vi "Get Channel Wise Calibration parameters.vi"(8 "error in (no error)":errorcluster, 10 "Physical Cgannel":string[](array[string]), 11 "Calibration Table":string[][](array[string])) -> (0 "error out":errorcluster, 2 "Array 2":sgl[][](array[numeric]), 3 "Slop & Offset":sgl[][](array[numeric]))   [LabVIEW 2018]
panel:
  out "subarray 2":string[](array[string])
  out "subarray":string[](array[string])
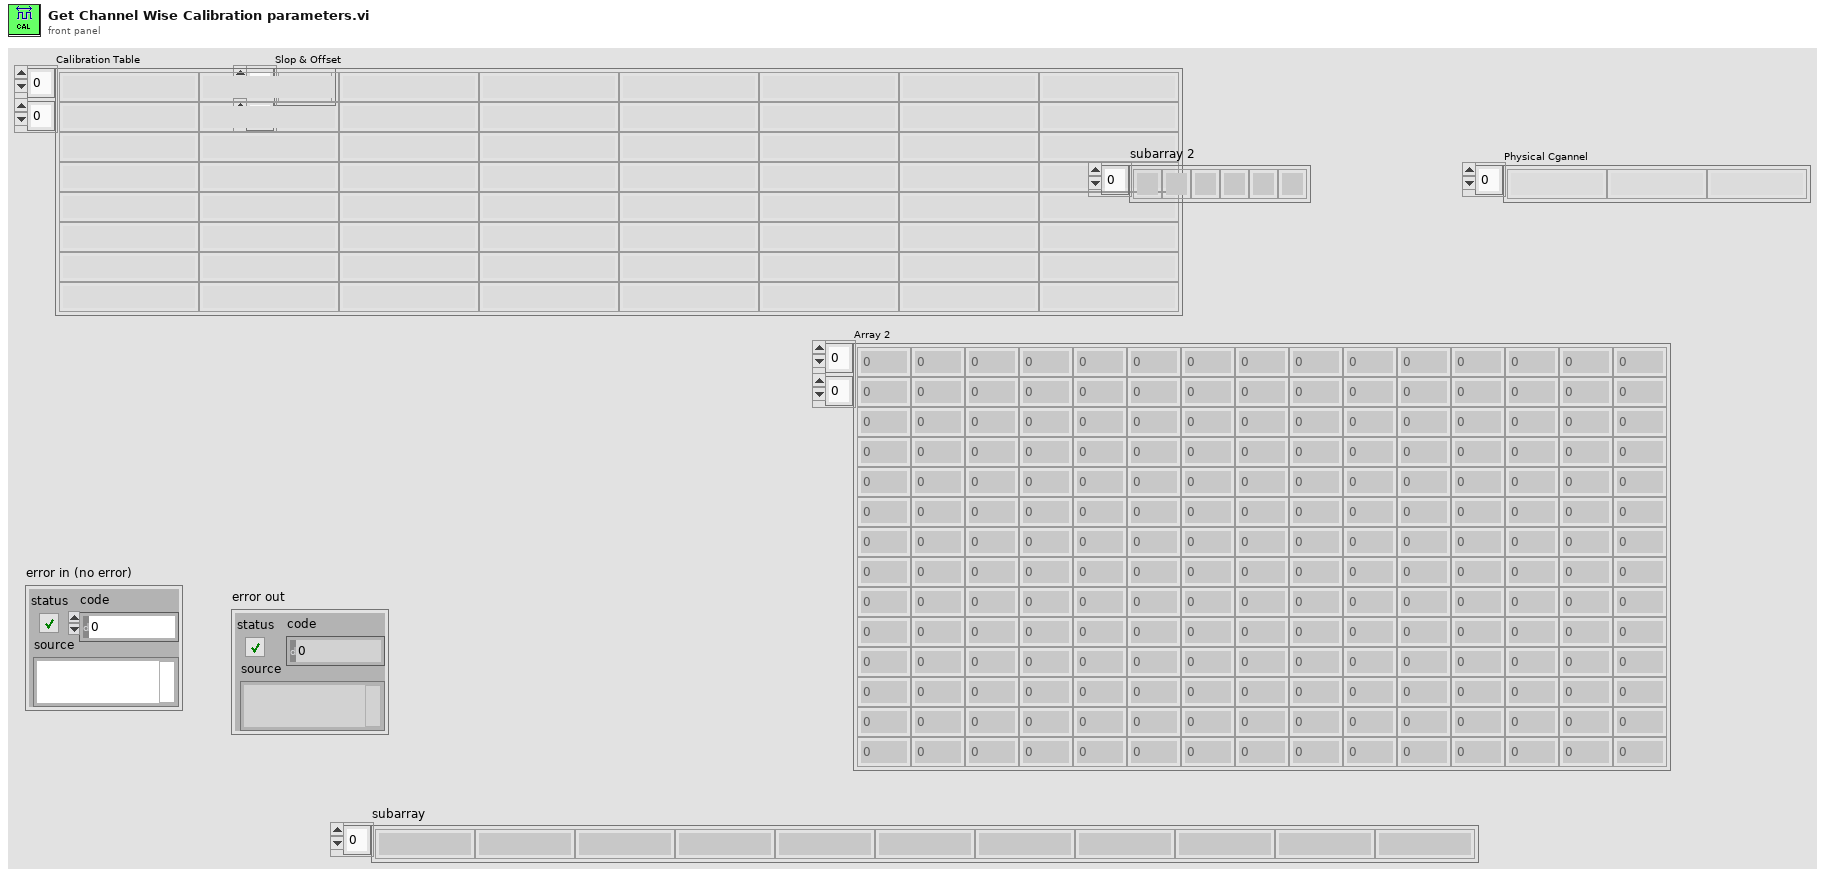
[diagram p1: front panel]
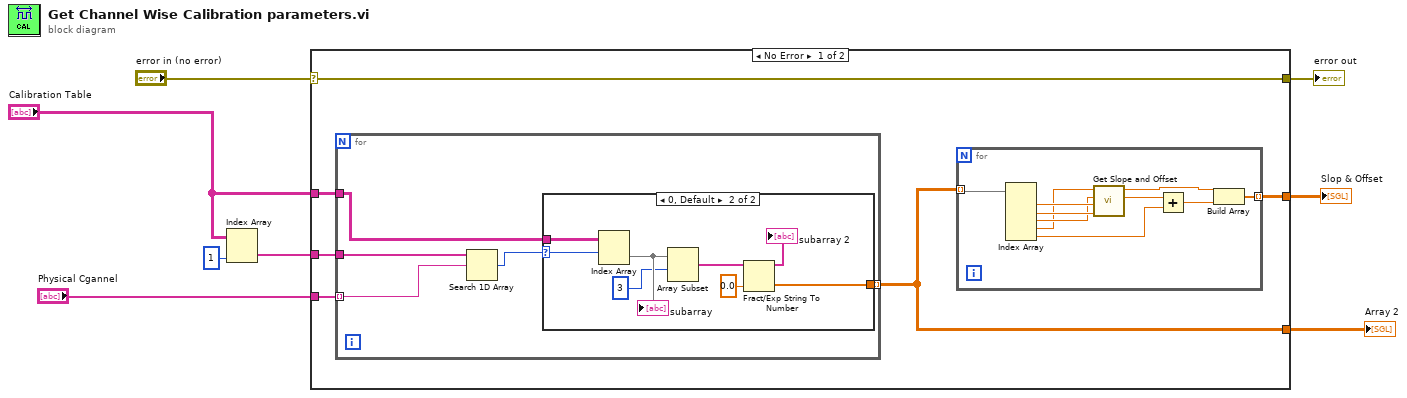
[diagram p0: block diagram]
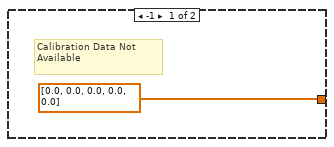
[diagram p2: hidden frame]
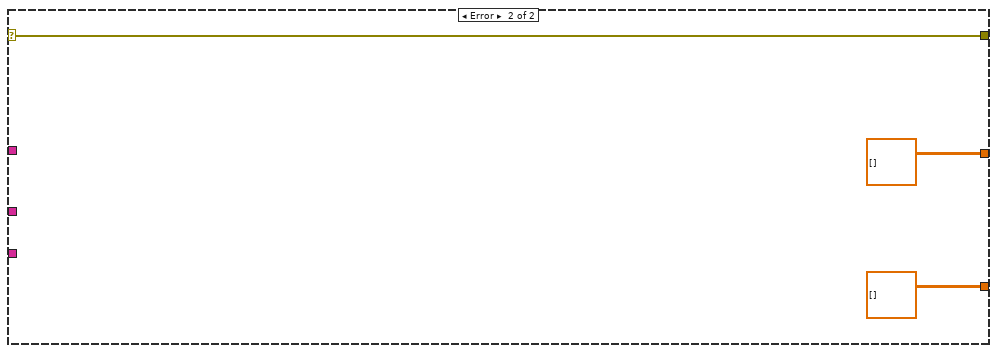
[diagram p3: hidden frame]
diagram:
  n1 = Index Array(array="Calibration Table", index (col)=1 ("disabled index (col)")) -> (element=w4:string[])  [unwired: 1 in]
  n2 = case shown="No Error" "error in (no error)" {
    selector: "error in (no error)" -> [w9 w38]
    tunnel: [w14 sgl[][] []] -> w8
    tunnel: [w13 sgl[][] [] ("Array")] -> w7
    tunnel: "Calibration Table" -> [w12 _]
    tunnel: "Physical Cgannel" -> [w11 _]
    tunnel: w4 -> [w10 _]
    tunnel: [w9 w38] -> w1
    frame No Error {
      n3 = for {
        tunnel: w10 -> [w29]
        tunnel: w11 -> [w28] mode=indexing
        tunnel: w12 -> [w27]
        tunnel: [w26] -> w13 mode=indexing
        n4 = Search 1D Array(1D array=w29, element=w28) -> (index of element=w25:i32)  [unwired: 1 in]
        n5 = case shown="0, Default" w25 {
          selector: w25 -> [_ w31]
          tunnel: w27 -> [_ w37]
          tunnel: [sgl[] [0.0, 0.0, 0.0, 0.0, 0.0] ("Array") w32] -> w26
          frame -1 {
            # "Calibration Data Not \nAvailable"
          }
          frame 0, Default {
            n6 = Index Array "Index Array"(array=w37, index (row)=w31) -> (element=w36:string[])  [unwired: 1 in]
            "subarray" <- w36
            n7 = Array Subset "Array Subset"(array=w36, index=3) -> (w34:string[])  [unwired: 1 in]
            "subarray 2" <- w34
            n8 = Fract/Exp String To Number(string=w34, default (0 dbl)=sgl 0.0 ("default (0 DBL)")) -> (number=w32:sgl[])  [unwired: 2 in, 1 out]
          }
        }
      }
      n9 = for {
        tunnel: w13 -> [w24] mode=indexing
        tunnel: [w15] -> w14 mode=indexing
        n10 = Index Array(array=w24) -> (element #1=w23:sgl, element #2=w22:sgl, element #3=w21:sgl, element #4=w20:sgl, element #5=w18:sgl)  [unwired: 5 in]
        n11 = call "Get Slope and Offset.vi"("raw max"=w22, "raw min"=w23, "emin"=w21, "emax"=w20) -> ("c"=w19:sgl, "m"=w17:sgl)  [unwired: 6 in]
        n12 = Add(x=w19, y=w18) -> (x+y=w16:sgl)
        n13 = Build Array(w17, w16) -> (w15:sgl[])
      }
    }
    frame Error {
    }
  }
  "Slop & Offset" <- w8
  "Array 2" <- w7
  "error out" <- w1
